vi "Extrae_SetField.vi"(10 "String":string="Set Magnetic Field 1000.000Tesla at 100.000Tesla/min, Linear, Persistent, Wait") -> (1 "Array":string[](array[string]))   [LabVIEW 2017]
panel:
  # "Set Magnetic Field 1000.000Tesla at 100.000Tesla/min, Linear, Persistent, Wait"
  # "Set Magnetic Field 1000.000Tesla at 100.000Tesla/min, Linear, Persistent, Sweep&meas"
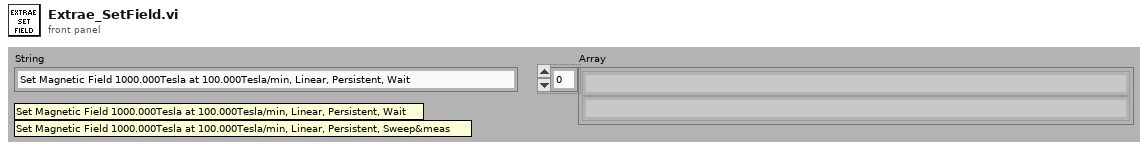
[diagram p1: front panel]
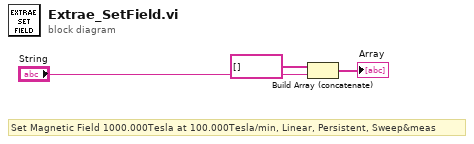
[diagram p0: block diagram]
diagram:
  # "Set Magnetic Field 1000.000Tesla at 100.000Tesla/min, Linear, Persistent, Sweep&meas"
  n1 = Build Array (concatenate)(string[] [] ("Array I"), "String") -> (→"Array":string[])
